vi "Query Scan Response Message.vi"(8 "error in":errorcluster, 10 "Error Query (Enabled)":bool=TRUE caption="Error Query", 11 "VISA resource name":refnum<visa-resource-name>) -> (0 "error out":errorcluster, 2 "Response Strings":string[](array[string]), 3 "VISA resource name out":refnum<visa-resource-name>)   [LabVIEW 2014, in "Hokuyo URG Series.lvlib"]
doc: "Reads the entire scan response string in continuous mode. This VI also checks the stats bit of the response for errors (if enabled) The scan response message has the same format as that of a response message."
uses:
  Hokuyo URG Series.lvlib
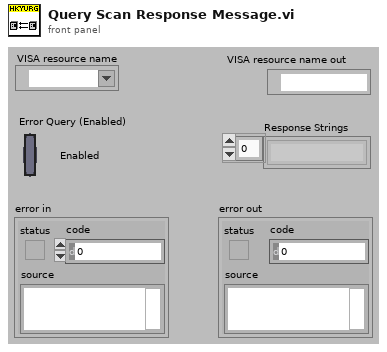
[diagram p1: front panel]
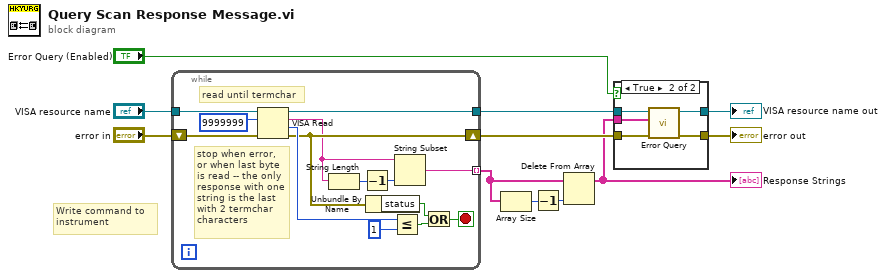
[diagram p0: block diagram]
diagram:
  # "Write command to\ninstrument"
  n1 = while {
    tunnel: "VISA resource name" -> [w17]
    shift-right: [w18] -> w5
    shift-left: "error in" -> [w20]
    tunnel: [w13] -> w9 mode=indexing
    tunnel: [w25] -> w7
    stop <- w22 stop-if-true
    # "stop when error, or when last byte is read -- the only response with one string is the last with 2 termchar characters"
    # "read until termchar"
    n2 = VISA Read(VISA resource name=w17, byte count=u32 9999999, error in (no error)=w20) -> (VISA resource name out=w25:refnum<visa-resource-name>, read buffer=w12:string, return count=w24:u32, error out=w18:errorcluster)
    n3 = String Length(string=w12) -> (length=w14:i32)
    n4 = Decrement(x=w14) -> (x-1=w15:i32)
    n5 = Unbundle By Name(w18) -> ("status"=w19:bool)
    n6 = Less Or Equal?(x=w24, y=u32 1) -> (x <= y?=w21:bool)
    n7 = String Subset(string=w12, length (rest)=w15) -> (substring=w13:string)  [unwired: 1 out]
    n8 = Or(x=w19, y=w21) -> (x .or. y?=w22:bool)
  }
  n9 = Array Size(array=w9) -> (size(s)=w11:i32)
  n10 = Decrement(x=w11) -> (x-1=w10:i32)
  n11 = Delete From Array(array=w9, index=w10) -> (array with subset deleted=w3:string[])  [unwired: 1 in, 1 out]
  "Response Strings" <- w3
  n12 = case shown="True" "Error Query (Enabled)" {
    tunnel: [w27 w31] -> w8
    tunnel: w7 -> [w27 w32]
    tunnel: w5 -> [w26 w30]
    tunnel: [w26 w29] -> w4
    tunnel: w3 -> [_ w28]
    frame False {
    }
    frame True {
      n13 = call "Error Query.vi"("error in (no error)"=w30, "Instrument Message"=w28, "VISA resource name"=w32) -> ("error out"=w29:errorcluster, "VISA resource out"=w31:refnum<visa-resource-name>)  [unwired: 5 in, 2 out]
    }
  }
  "error out" <- w4
  "VISA resource name out" <- w8
